vi "Sea-Level SWI Preset.vi"(7 "Sea-Level SWI":T2, 8 "error in (no error)":errorcluster, 11 "Handle":i32) -> (0 "error out":errorcluster, 3 "Handle Out":i32, 5 "SWI Position":T1)   [LabVIEW 2011]
uses:
  TypeDefs/Sea-Level SWI Adapter Info.ctl
  TypeDefs/Sea-Level SWI Position.ctl
  TypeDefs/Sea-Level SWI Access Mode.ctl
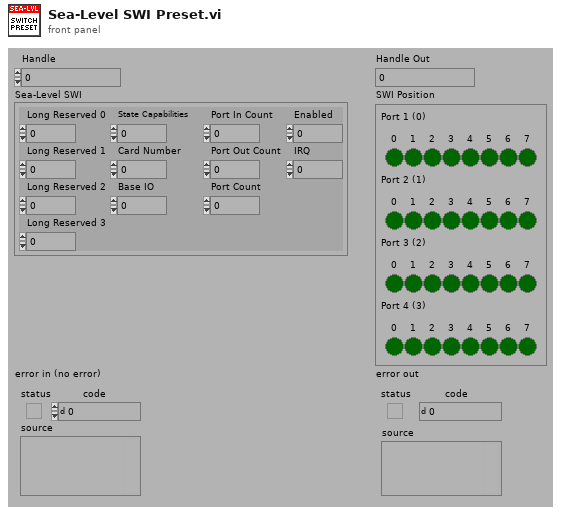
[diagram p1: front panel]
types:
  T1 = typedef "Sea-Level SWI Position.ctl" = cluster{"Port 1 (0)":cluster{"0":bool, "1":bool, "2":bool, "3":bool, "4":bool, "5":bool, "6":bool, "7":bool}, "Port 2 (1)":cluster{"0":bool, "1":bool, "2":bool, "3":bool, "4":bool, "5":bool, "6":bool, "7":bool}, "Port 3 (2)":cluster{"0":bool, "1":bool, "2":bool, "3":bool, "4":bool, "5":bool, "6":bool, "7":bool}, "Port 4 (3)":cluster{"0":bool, "1":bool, "2":bool, "3":bool, "4":bool, "5":bool, "6":bool, "7":bool}}
  T2 = typedef "Sea-Level SWI Adapter Info.ctl" = cluster{"Long Reserved 0":i32, "Long Reserved 1":i32, "Long Reserved 2":i32, "Long Reserved 3":i32, "State Capabilities":i32, "Card Number":i16, "Base IO":i16, "Port In Count":i8, "Port Out Count":i8, "Port Count":i8, "Enabled":i8, "IRQ":i16}
  T3 = typedef "Sea-Level SWI Access Mode.ctl" = enum16{"Relative", "Absolute"}
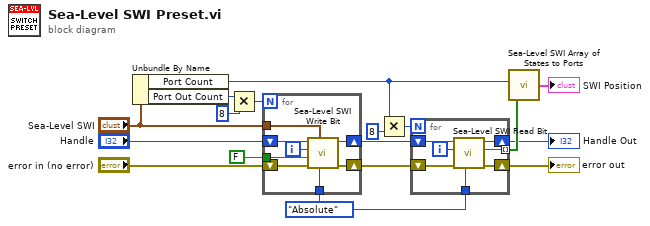
[diagram p0: block diagram]
diagram:
  w2 = Sea-Level_SWI_Access_Mode."Absolute" ("Access Mode (Relative)")
  n1 = Unbundle By Name("Sea-Level SWI") -> ("Port Count"=w1:i8, "Port Out Count"=w13:i8)
  n2 = Multiply(x=w13, y=i8 8) -> (x*y=w11:i8)
  n3 = for {
    N: w11 -> [_]
    tunnel: "Sea-Level SWI" -> [w21]
    tunnel: FALSE ("State") -> [w20]
    tunnel: w2 -> [w19]
    shift-right: [w23] -> w6
    shift-left: "Handle" -> [w22]
    shift-right: [w24] -> w5
    shift-left: "error in (no error)" -> [w25]
    i -> [w18]
    n4 = call "Sea-Level SWI Write Bit.vi"("Access Mode (Relative)"=w19, "Adapter Info"=w21, "error in (no error)"=w25, "State"=w20, "Bit Number"=w18, "Handle"=w22) -> ("error out"=w24:errorcluster, "Handle Out"=w23:i32)  [unwired: 4 out]
  }
  n5 = Multiply(x=w1, y=u32 8) -> (x*y=w9:u32)
  n6 = for {
    N: w9 -> [_]
    tunnel: [w27] -> w8 mode=indexing
    tunnel: w2 -> [w26]
    shift-right: [w30] -> w3
    shift-left: w6 -> [w31]
    shift-right: [w29] -> w4
    shift-left: w5 -> [w32]
    i -> [w28]
    n7 = call "Sea-Level SWI Read Bit.vi"("Access Mode (Relative)"=w26, "error in (no error)"=w32, "Bit Number"=w28, "Handle"=w31) -> ("error out"=w29:errorcluster, "State"=w27:bool, "Handle Out"=w30:i32)  [unwired: 1 in, 4 out]
  }
  "error out" <- w4
  "Handle Out" <- w3
  n8 = call "Sea-Level SWI Array of States to Ports.vi"("State Array"=w8, "Number of Ports"=w1) -> ("SWI Position"=→"SWI Position":T1)  [unwired: 2 out]
